vi "apply_offset_and_range.vi"(4 "colour below":u32(colorbox)=16860, 5 "colour above":u32(colorbox)=16711680, 6 "colour values below?":bool, 7 "colour values above?":bool, 8 "error in (no error)":errorcluster, 9 "range":dbl, 10 "offset":dbl, 11 "Image in":refnum<class "Image.lvclass">) -> (0 "error out":errorcluster, 3 "Image out":refnum<class "Image.lvclass">)   [LabVIEW 2010, in "Image.lvclass"]
uses:
  Image.lvclass
  comparison_operator_enum.ctl
  storage_mode.ctl
  ErrorController/ErrorController/class_data.vi
  <vilib>/vision/NI_Vision_Development_Module.lvlib
  ErrorController/ErrorController/ErrorController.lvclass
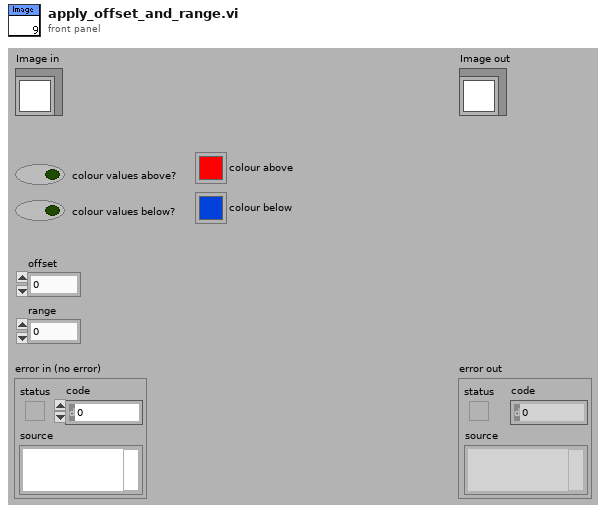
[diagram p1: front panel]
types:
  T1 = typedef "comparison_operator_enum.ctl" = enum16{"clear", "<", "=<", ">", "=>", "="}
  T2 = enum32{"Average", "Min", "Max", "Clear  if < ", "Clear  if < or =", "Clear  if =", "Clear  if > or =", "Clear  if >"}
  T3 = typedef "Image.lvclass/storage_mode.ctl" = enum16{"RAM", "disk"}
  T4 = typedef "IMAQ Image.ctl" = refnum<image>
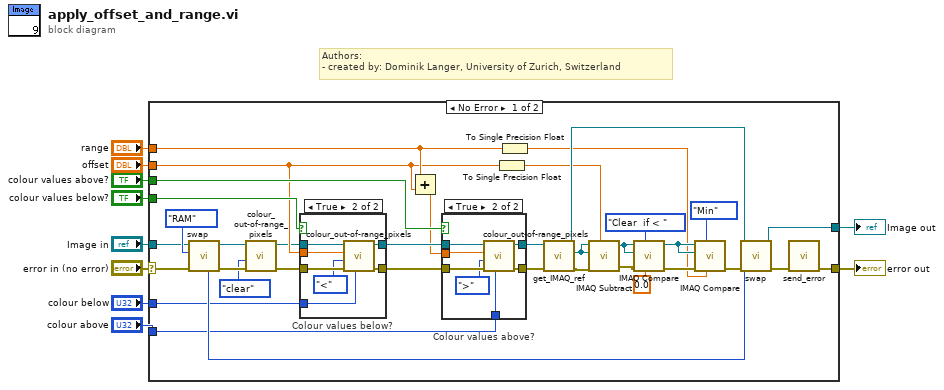
[diagram p0: block diagram]
diagram:
  # "Authors: \n- created by: Dominik Langer, University of Zurich, Switzerland"
  n1 = case shown="No Error" "error in (no error)" {
    selector: "error in (no error)" -> [w45 w66]
    tunnel: [w11 w66] -> w9
    tunnel: [w41 w65] -> w7
    tunnel: "Image in" -> [w43 w65]
    tunnel: "offset" -> [w19 _]
    tunnel: "range" -> [w21 _]
    tunnel: "colour values below?" -> [w24 _]
    tunnel: "colour above" -> [w29 _]
    tunnel: "colour values above?" -> [w23 _]
    tunnel: "colour below" -> [w30 _]
    frame No Error {
      n2 = call-dynamic "swap.vi"("error in (no error)"=w45, "storage type target"=storage_mode."RAM", "Image in"=w43) -> ("error out"=w15:errorcluster, "Image out"=w17:refnum<class "Image.lvclass">, "previous storage mode"=w42:T3)  [unwired: 6 out]
      n3 = call-dynamic "colour_out-of-range_pixels.vi"("error in (no error)"=w15, "comparison operator"=comparison_operator_enum."clear", "Image in"=w17) -> ("error out"=w14:errorcluster, "Image out"=w16:refnum<class "Image.lvclass">)  [unwired: 7 in]
      n4 = case "Colour values below?" shown="True" w24 {
        tunnel: w14 -> [w56 w64]
        tunnel: w16 -> [w57 w63]
        tunnel: w19 -> [_ w62]
        tunnel: w30 -> [_ w61]
        tunnel: [w57 w60] -> w28
        tunnel: [w56 w59] -> w26
        frame False {
        }
        frame True {
          n5 = call-dynamic "colour_out-of-range_pixels.vi"("colour"=w61, "error in (no error)"=w64, "comparison operator"=comparison_operator_enum."<", "comparison value"=w62, "Image in"=w63) -> ("error out"=w59:errorcluster, "Image out"=w60:refnum<class "Image.lvclass">)  [unwired: 5 in]
        }
      }
      n6 = Add(x=w21, y=w19) -> (x+y=w22:dbl)
      n7 = case "Colour values above?" shown="True" w23 {
        tunnel: w29 -> [_ w55]
        tunnel: w28 -> [w47 w54]
        tunnel: [w47 w53] -> w27
        tunnel: w26 -> [w48 w52]
        tunnel: [w48 w51] -> w25
        tunnel: w22 -> [_ w50]
        frame False {
        }
        frame True {
          n8 = call-dynamic "colour_out-of-range_pixels.vi"("colour"=w55, "error in (no error)"=w52, "comparison operator"=comparison_operator_enum.">", "comparison value"=w50, "Image in"=w54) -> ("error out"=w51:errorcluster, "Image out"=w53:refnum<class "Image.lvclass">)  [unwired: 5 in]
        }
      }
      n9 = To Single Precision Float(number=w19) -> (single precision float=w18:sgl)
      n10 = To Single Precision Float(number=w21) -> (single precision float=w20:sgl)
      n11 = call-dynamic "get_IMAQ_ref.vi"("error in (no error)"=w25, "Image.lvclass in"=w27) -> ("error out"=w33:errorcluster, "Image"=w34:T4, "Image.lvclass out"=w32:refnum<class "Image.lvclass">)  [unwired: 7 out]
      n12 = call "IMAQ Subtract"("Image Src A"=w34, "Constant"=w18, "Image Dst"=w34, "error in (no error)"=w33) -> ("Image Dst Out"=w36:T4, "error out"=w39:errorcluster)  [unwired: 1 in, 2 out]
      n13 = call "IMAQ Compare"("Constant"=sgl 0.0, "Operator"=T2."Clear  if < ", "error in (no error)"=w39, "Image Dst"=w36, "Image Src A"=w36) -> ("error out"=w38:errorcluster, "Image Dst Out"=w35:T4)  [unwired: 1 in, 4 out]
      n14 = call "IMAQ Compare"("Constant"=w20, "Operator"=T2."Min", "error in (no error)"=w38, "Image Dst"=w35, "Image Src A"=w35) -> ("error out"=w31:errorcluster)  [unwired: 1 in, 5 out]
      n15 = call-dynamic "swap.vi"("error in (no error)"=w31, "storage type target"=w42, "Image in"=w32) -> ("error out"=w12:errorcluster, "Image out"=w41:refnum<class "Image.lvclass">)  [unwired: 7 out]
      n16 = call "send_error.vi"("error in (no error)"=w12) -> ("error out"=w11:errorcluster)  [unwired: 10 in]
    }
    frame Error {
    }
  }
  "error out" <- w9
  "Image out" <- w7
